vi "array sizes to number of points.vi"(11 "Size(s)":i32[](array[numeric])) -> (3 "#scalar values":i32)   [LabVIEW 2021, in "Ring Buffer Strict Accessor.lvlib"]
uses:
  Ring Buffer Strict Accessor.lvlib
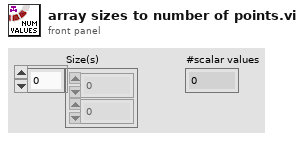
[diagram p1: front panel]
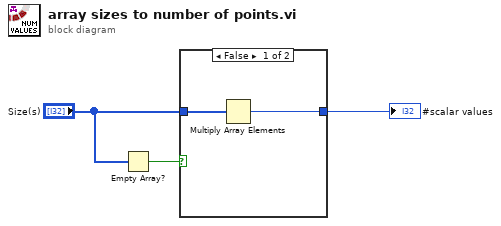
[diagram p0: block diagram]
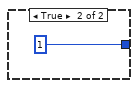
[diagram p2: hidden frame]
diagram:
  n1 = Empty Array?(array="Size(s)") -> (empty?=w3:bool)
  n2 = case shown="False" w3 {
    tunnel: "Size(s)" -> [w5 _]
    tunnel: [w4 1 ("Size(s)")] -> w1
    frame False {
      n3 = Multiply Array Elements(1:w5) -> (0:w4:i32)
    }
    frame True {
    }
  }
  "#scalar values" <- w1
